vi "DIO card.vi"(8 "error in (no error)":errorcluster, 11 "Node Ptr":T4 format="%.0x") -> (0 "error out":errorcluster)   [LabVIEW 2014, in "SLSC configuration System Explorer.lvlib"]
uses:
  SLSC configuration System Explorer.lvlib
  <vilib>/NI Veristand/Custom Device API/Custom Device Item Ref.ctl
  Example/DIO Board/DIO Line Config.ctl
  Type Defs/Card Position.ctl
  Example/SPI Utility/Slot #.ctl
  Shared/Constants.vi
  <vilib>/NI Veristand/Custom Device API/Get Item Property (U16).vi
  <vilib>/NI Veristand/Custom Device API/Set Item Property (U16).vi
  <vilib>/NI Veristand/Custom Device API/Custom Device API.lvlib
  Shared/SLSC configuration Shared.lvlib
panel:
  in  "Card Position":T1 {"Slot #" max=16}
  in  "Logic Threshold (%) 3":u8 caption="Logic Threshold (%)"
  in  "DIO Line Config 3":T3=[FALSE, FALSE, FALSE, FALSE, FALSE, FALSE, FALSE, FALSE]
  in  "Header 5":cluster{"Section Name":string}={"Section Name"="Bank 3 Settings"}
  in  "Logic Threshold (%) 2":u8 caption="Logic Threshold (%)"
  in  "DIO Line Config 2":T3=[FALSE, FALSE, FALSE, FALSE, FALSE, FALSE, FALSE, FALSE]
  in  "Header 4":cluster{"Section Name":string}={"Section Name"="Bank 2 Settings"}
  in  "Header 3":cluster{"Section Name":string}={"Section Name"="Bank 1 Settings"}
  in  "Logic Threshold (%) 1":u8 caption="Logic Threshold (%)"
  in  "DIO Line Config 1":T3=[FALSE, FALSE, FALSE, FALSE, FALSE, FALSE, FALSE, FALSE]
  in  "Header 2":cluster{"Section Name":string}={"Section Name"="Bank 0 Settings"}
  in  "Logic Threshold (%) 0":u8 caption="Logic Threshold (%)"
  in  "DIO Line Config 0":T3=[FALSE, FALSE, FALSE, FALSE, FALSE, FALSE, FALSE, FALSE]
  in  "Header":cluster{"Section Name":string}={"Section Name"="DIO Card Settings"}
  in  "Description":string
  in  "Name":string
  # "Line 9"
  # "Line 10"
  # "Line 11"
  # "Line 12"
  # "Line 13"
  # "Line 14"
  # "Line 15"
  # "Line 16"
  # "Line 17"
  # "Line 18"
  # "Line 19"
  # "Line 20"
  # "Line 21"
  # "Line 22"
  # "Line 23"
  # "Line 24"
  # "Line 25"
  # "Line 26"
  # "Line 27"
  # "Line 28"
  # "Line 29"
  # "Line 30"
  # "Line 31"
  # "Line 32"
  # "Line 1"
  # "Line 2"
  # "Line 3"
  # "Line 4"
  # "Line 5"
  # "Line 6"
  # "Line 7"
  # "Line 8"
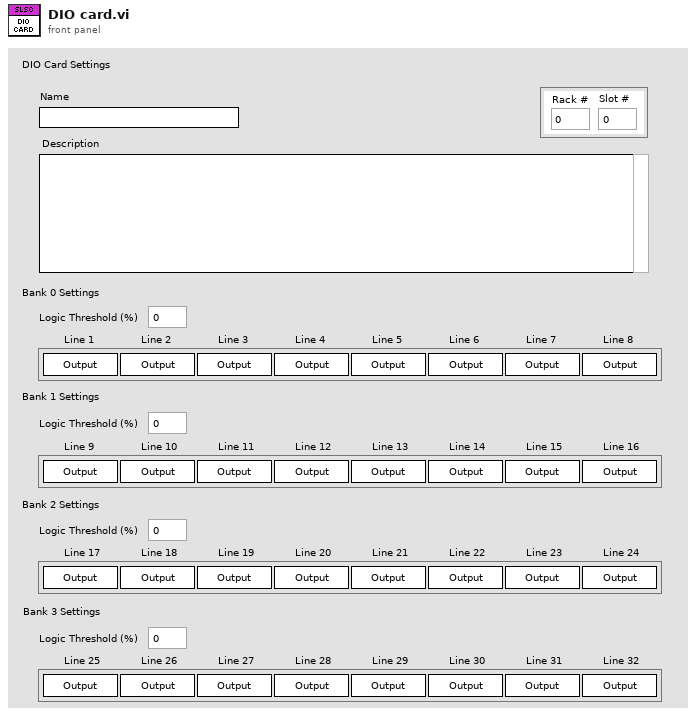
[diagram p1: front panel]
types:
  T1 = typedef "SLSC configuration Shared.lvlib/Card Position.ctl" = cluster{"Rack #":u8, "Slot #":T2}
  T2 = typedef "SLSC configuration Shared.lvlib/Slot #.ctl" = u8
  T3 = typedef "SLSC configuration Shared.lvlib/DIO Line Config.ctl" = bool[]
  T4 = typedef "Custom Device API.lvlib/Custom Device Item Ref.ctl" = u64
  T5 = typedef "Custom Device API.lvlib/Custom Device Commands.ctl" = enum16{"Default", "Item renamed", "Shutdown", "Dynamic button pressed"}
  T6 = typedef "Custom Device API.lvlib/Custom Device Item Info.ctl" = cluster{"Name":string, "Is Channel":bool, "GUID":string, "Is Waveform":bool}
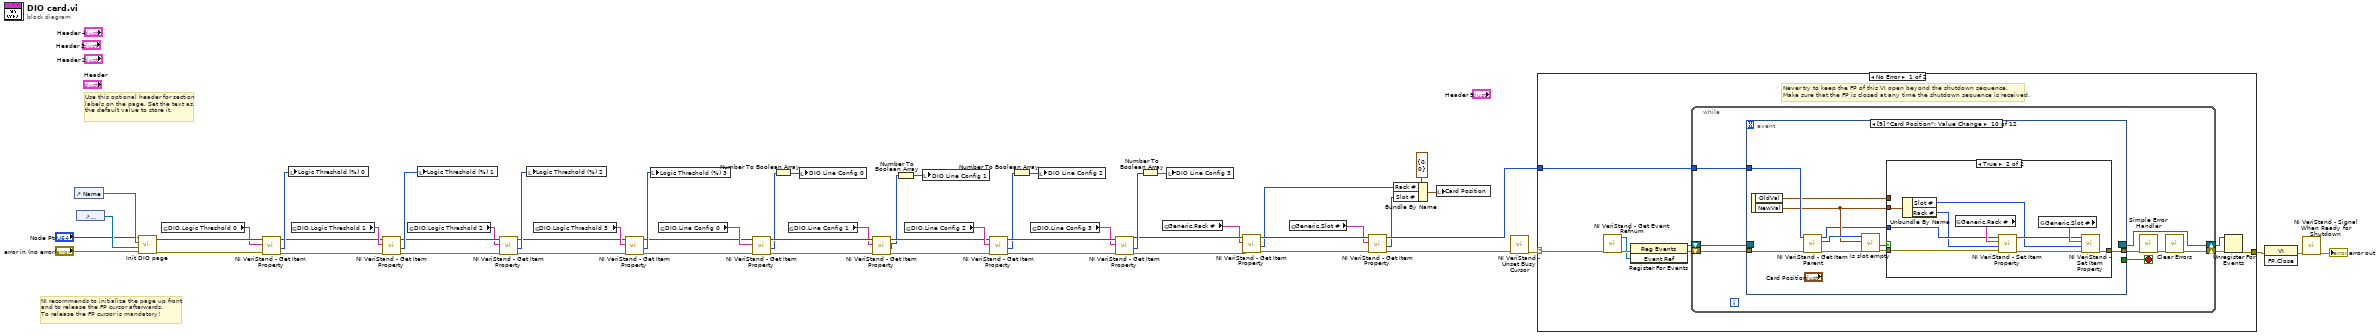
[diagram p0: block diagram]
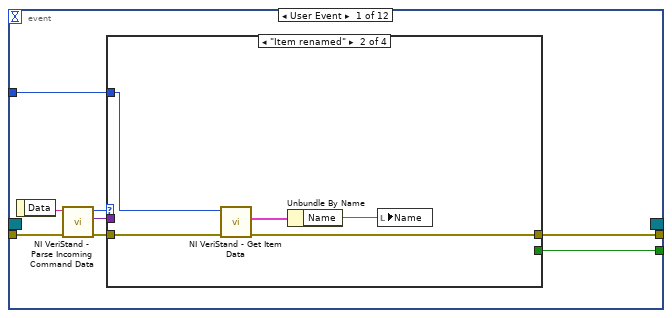
[diagram p2: hidden frame]
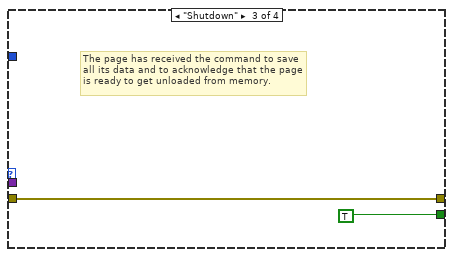
[diagram p4: hidden frame]
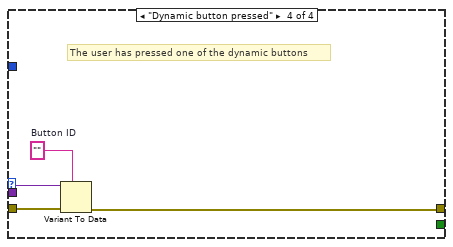
[diagram p5: hidden frame]
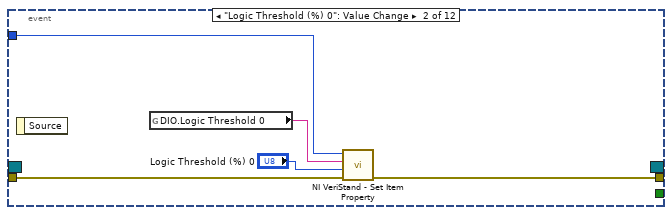
[diagram p6: hidden frame]
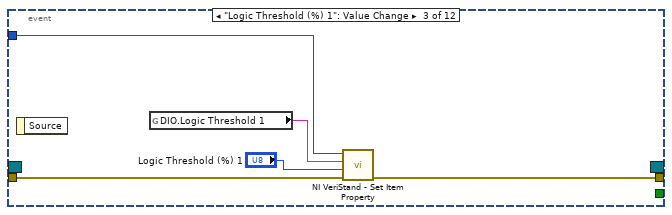
[diagram p7: hidden frame]
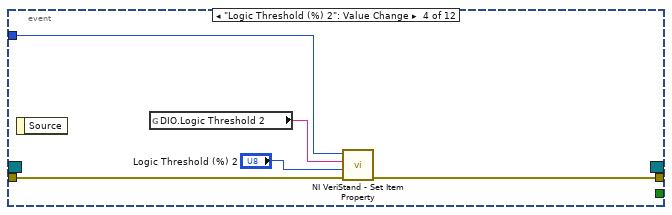
[diagram p8: hidden frame]
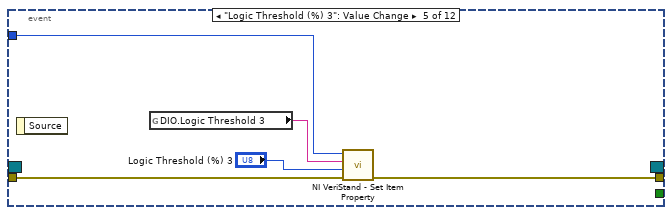
[diagram p9: hidden frame]
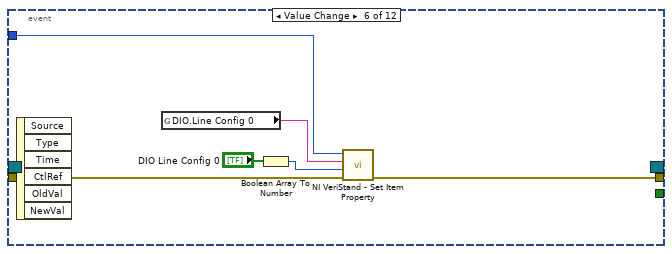
[diagram p10: hidden frame]
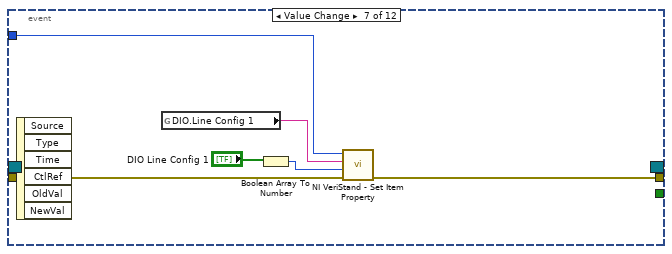
[diagram p11: hidden frame]
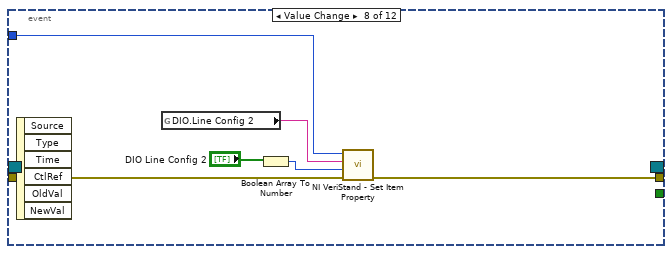
[diagram p12: hidden frame]
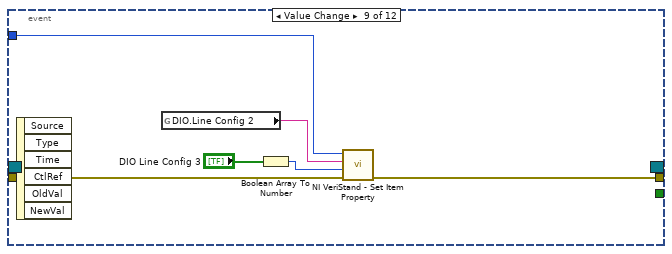
[diagram p13: hidden frame]
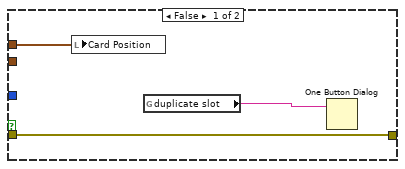
[diagram p14: hidden frame]
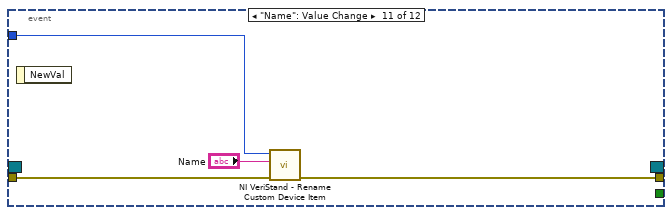
[diagram p15: hidden frame]
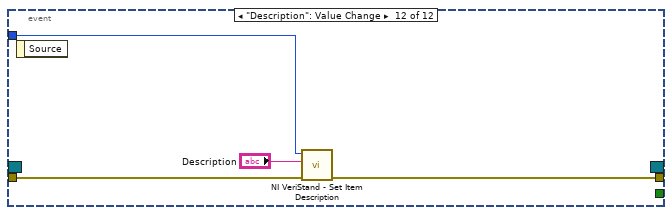
[diagram p16: hidden frame]
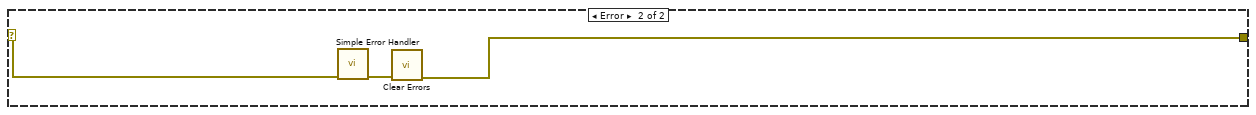
[diagram p17: hidden frame]
diagram:
  # "Use this optional header for section labels on the page. Set the text as the default value to store it."
  # "NI recommends to initialize the page up front\nand to release the FP cursor afterwards.\nTo release the FP cursor is mandatory!"
  n1 = control-ref of="Name"() -> (w52:refnum<vi>)
  n2 = control-ref of="Description"() -> (w51:refnum<vi>)
  n3 = call "Init DIO page.vi"("error in (no error)"="error in (no error)", "Description"=w51, "Name"=w52, "Node Ptr"="Node Ptr") -> ("error out"=w48:errorcluster, "Node Ptr out"=w47:T4)  [unwired: 6 in]
  n4 = global read "Constants.vi" "DIO.Logic Threshold 0"() -> (w45:string)
  n5 = call-poly <vilib>:"NI VeriStand - Get Item Property.vi"("error in (no error)"=w48, "Property Name"=w45, "Item Ref in"=w47) -> ("error out"=w42:errorcluster, "Value"=w46:u16, "Item Ref out"=w41:T4)  [unwired: 5 in, 1 out]
  n6 = local write "Logic Threshold (%) 0"(w46) -> ()
  n7 = global read "Constants.vi" "DIO.Logic Threshold 1"() -> (w44:string)
  n8 = call-poly <vilib>:"NI VeriStand - Get Item Property.vi"("error in (no error)"=w42, "Property Name"=w44, "Item Ref in"=w41) -> ("error out"=w39:errorcluster, "Value"=w43:u16, "Item Ref out"=w38:T4)  [unwired: 5 in, 1 out]
  n9 = global read "Constants.vi" "DIO.Logic Threshold 2"() -> (w37:string)
  n10 = local write "Logic Threshold (%) 1"(w43) -> ()
  n11 = call-poly <vilib>:"NI VeriStand - Get Item Property.vi"("error in (no error)"=w39, "Property Name"=w37, "Item Ref in"=w38) -> ("error out"=w34:errorcluster, "Value"=w40:u16, "Item Ref out"=w33:T4)  [unwired: 5 in, 1 out]
  n12 = local write "Logic Threshold (%) 2"(w40) -> ()
  n13 = global read "Constants.vi" "DIO.Logic Threshold 3"() -> (w36:string)
  n14 = call-poly <vilib>:"NI VeriStand - Get Item Property.vi"("error in (no error)"=w34, "Property Name"=w36, "Item Ref in"=w33) -> ("error out"=w21:errorcluster, "Value"=w35:u16, "Item Ref out"=w20:T4)  [unwired: 5 in, 1 out]
  n15 = local write "Logic Threshold (%) 3"(w35) -> ()
  n16 = global read "Constants.vi" "DIO.Line Config 0"() -> (w23:string)
  n17 = call-poly <vilib>:"NI VeriStand - Get Item Property.vi"("error in (no error)"=w21, "Property Name"=w23, "Item Ref in"=w20) -> ("error out"=w25:errorcluster, "Value"=w22:u16, "Item Ref out"=w26:T4)  [unwired: 5 in, 1 out]
  n18 = Number To Boolean Array(number=w22) -> (Boolean array=w19:bool[])
  n19 = global read "Constants.vi" "DIO.Line Config 1"() -> (w24:string)
  n20 = local write "DIO Line Config 0"(w19) -> ()
  n21 = call-poly <vilib>:"NI VeriStand - Get Item Property.vi"("error in (no error)"=w25, "Property Name"=w24, "Item Ref in"=w26) -> ("error out"=w27:errorcluster, "Value"=w17:u16, "Item Ref out"=w28:T4)  [unwired: 5 in, 1 out]
  n22 = Number To Boolean Array(number=w17) -> (Boolean array=w18:bool[])
  n23 = global read "Constants.vi" "DIO.Line Config 2"() -> (w29:string)
  n24 = local write "DIO Line Config 1"(w18) -> ()
  n25 = call-poly <vilib>:"NI VeriStand - Get Item Property.vi"("error in (no error)"=w27, "Property Name"=w29, "Item Ref in"=w28) -> ("error out"=w31:errorcluster, "Value"=w15:u16, "Item Ref out"=w32:T4)  [unwired: 5 in, 1 out]
  n26 = Number To Boolean Array(number=w15) -> (Boolean array=w16:bool[])
  n27 = global read "Constants.vi" "DIO.Line Config 3"() -> (w30:string)
  n28 = local write "DIO Line Config 2"(w16) -> ()
  n29 = call-poly <vilib>:"NI VeriStand - Get Item Property.vi"("error in (no error)"=w31, "Property Name"=w30, "Item Ref in"=w32) -> ("error out"=w9:errorcluster, "Value"=w13:u16, "Item Ref out"=w8:T4)  [unwired: 5 in, 1 out]
  n30 = Number To Boolean Array(number=w13) -> (Boolean array=w14:bool[])
  n31 = global read "Constants.vi" "Generic.Rack #"() -> (w7:string)
  n32 = local write "DIO Line Config 3"(w14) -> ()
  n33 = call-poly <vilib>:"NI VeriStand - Get Item Property.vi"("error in (no error)"=w9, "Property Name"=w7, "Item Ref in"=w8) -> ("error out"=w11:errorcluster, "Value"=w3:u16, "Item Ref out"=w12:T4)  [unwired: 5 in, 1 out]
  n34 = global read "Constants.vi" "Generic.Slot #"() -> (w10:string)
  n35 = call-poly <vilib>:"NI VeriStand - Get Item Property.vi"("error in (no error)"=w11, "Property Name"=w10, "Item Ref in"=w12) -> ("error out"=w6:errorcluster, "Value"=w2:u16, "Item Ref out"=w5:T4)  [unwired: 5 in, 1 out]
  n36 = Bundle By Name(cluster=T1 {"Rack #"=0, "Slot #"=0} ("Card Position"), "Rack #"=w3, "Slot #"=w2) -> (w1:T1)
  n37 = local write "Card Position"(w1) -> ()
  n38 = call <vilib>:"NI VeriStand - Unset Busy Cursor.vi"("error in (no error)"=w6) -> ("error out"=w53:errorcluster)  [unwired: 10 out]
  n39 = case shown="No Error" w53 {
    selector: w53 -> [w58 w171]
    tunnel: [w62 w169] -> w56
    tunnel: w5 -> [w57 _]
    frame No Error {
      # "Never try to keep the FP of this VI open beyond the shutdown sequence.\nMake sure that the FP is closed at any time the shutdown sequence is received."
      n40 = call <vilib>:"NI VeriStand - Get Event Refnum.vi"("error in (no error)"=w58) -> ("error out"=w65:errorcluster, "Event Ref"=w61:refnum<user-event>)  [unwired: 9 out]
      n41 = register-events(error in=w65, w61) -> (reference out=w59:refnum<event-registration>, error out=w60:errorcluster)  [unwired: 1 in]
      n42 = while {
        shift-right: [w67] -> w63
        shift-left: w60 -> [w72]
        shift-right: [w73] -> w64
        shift-left: w59 -> [w71]
        tunnel: w57 -> [w66]
        stop <- w70 stop-if-true
        n43 = event shown="[9] \"Card Position\": Value Change" {
          selector: w71 -> [_ _ _ _ _ _ _ _ _ _ _ _]
          dyn-events: [_ _ _ _ _ _ _ _ _ _ _ _] -> w73
          timeout: _ -> [_ _ _ _ _ _ _ _ _ _ _ _]
          tunnel: w72 -> [w81 w98 w103 w108 w113 w119 w125 w131 w137 w146 w164 w168]
          tunnel: [w77 _ _ _ _ _ _ _ _ _ _ _] -> w70
          tunnel: [w76 w97 w102 w107 w112 w118 w124 w130 w136 w147 w163 w167] -> w69
          tunnel: w66 -> [w74 w94 w99 w104 w109 w114 w120 w126 w132 w145 w161 w165]
          event User Event {
            n44 = event-data() -> ("Data"=w80:string)  [unwired: 1 out]
            n45 = call <vilib>:"NI VeriStand - Parse Incoming Command Data.vi"("error in (no error)"=w81, "Incoming data"=w80) -> ("error out"=w79:errorcluster, "Outgoing data"=w75:variant, "Action"=w78:T5)  [unwired: 7 out]
            n46 = case shown="\"Item renamed\"" w78 {
              tunnel: w79 -> [w82 w87 w88 w93]
              tunnel: [_ _ TRUE _] -> w77
              tunnel: [w82 w85 w88 w90] -> w76
              tunnel: w75 -> [_ _ _ w92]
              tunnel: w74 -> [_ w83 _ _]
              frame "Default", Default {
              }
              frame "Item renamed" {
                n47 = call <vilib>:"NI VeriStand - Get Item Data.vi"("error in (no error)"=w87, "Item Ref in"=w83) -> ("error out"=w85:errorcluster, "Item Info"=w86:T6)  [unwired: 8 out]
                n48 = Unbundle By Name(w86) -> ("Name"=w84:string)
                n49 = local write "Name"(w84) -> ()
              }
              frame "Shutdown" {
                # "The page has received the command to save all its data and to acknowledge that the page is ready to get unloaded from memory."
              }
              frame "Dynamic button pressed" {
                w91 = ""  # Button ID
                # "The user has pressed one of the dynamic buttons"
                n50 = Variant To Data(error in=w93, type=w91, Variant=w92) -> (error out=w90:errorcluster)  [unwired: 1 out]
              }
            }
          }
          event "Logic Threshold (%) 0": Value Change {
            n51 = event-data() -> ()  [unwired: 2 out]
            n52 = global read "Constants.vi" "DIO.Logic Threshold 0"() -> (w95:string)
            n53 = call-poly <vilib>:"NI VeriStand - Set Item Property.vi"("error in (no error)"=w98, "Value"="Logic Threshold (%) 0", "Property Name"=w95, "Item Ref in"=w94) -> ("error out"=w97:errorcluster)  [unwired: 5 in, 2 out]
          }
          event "Logic Threshold (%) 1": Value Change {
            n54 = event-data() -> ()  [unwired: 2 out]
            n55 = global read "Constants.vi" "DIO.Logic Threshold 1"() -> (w101:string)
            n56 = call-poly <vilib>:"NI VeriStand - Set Item Property.vi"("error in (no error)"=w103, "Value"="Logic Threshold (%) 1", "Property Name"=w101, "Item Ref in"=w99) -> ("error out"=w102:errorcluster)  [unwired: 5 in, 2 out]
          }
          event "Logic Threshold (%) 2": Value Change {
            n57 = event-data() -> ()  [unwired: 2 out]
            n58 = global read "Constants.vi" "DIO.Logic Threshold 2"() -> (w106:string)
            n59 = call-poly <vilib>:"NI VeriStand - Set Item Property.vi"("error in (no error)"=w108, "Value"="Logic Threshold (%) 2", "Property Name"=w106, "Item Ref in"=w104) -> ("error out"=w107:errorcluster)  [unwired: 5 in, 2 out]
          }
          event "Logic Threshold (%) 3": Value Change {
            n60 = event-data() -> ()  [unwired: 2 out]
            n61 = global read "Constants.vi" "DIO.Logic Threshold 3"() -> (w111:string)
            n62 = call-poly <vilib>:"NI VeriStand - Set Item Property.vi"("error in (no error)"=w113, "Value"="Logic Threshold (%) 3", "Property Name"=w111, "Item Ref in"=w109) -> ("error out"=w112:errorcluster)  [unwired: 5 in, 2 out]
          }
          event Value Change {
            n63 = event-data() -> ()  [unwired: 7 out]
            n64 = global read "Constants.vi" "DIO.Line Config 0"() -> (w117:string)
            n65 = Boolean Array To Number(Boolean array="DIO Line Config 0") -> (number=w115:u8)
            n66 = call-poly <vilib>:"NI VeriStand - Set Item Property.vi"("error in (no error)"=w119, "Value"=w115, "Property Name"=w117, "Item Ref in"=w114) -> ("error out"=w118:errorcluster)  [unwired: 5 in, 2 out]
          }
          event Value Change {
            n67 = event-data() -> ()  [unwired: 7 out]
            n68 = global read "Constants.vi" "DIO.Line Config 1"() -> (w123:string)
            n69 = Boolean Array To Number(Boolean array="DIO Line Config 1") -> (number=w122:u8)
            n70 = call-poly <vilib>:"NI VeriStand - Set Item Property.vi"("error in (no error)"=w125, "Value"=w122, "Property Name"=w123, "Item Ref in"=w120) -> ("error out"=w124:errorcluster)  [unwired: 5 in, 2 out]
          }
          event Value Change {
            n71 = event-data() -> ()  [unwired: 7 out]
            n72 = global read "Constants.vi" "DIO.Line Config 2"() -> (w129:string)
            n73 = Boolean Array To Number(Boolean array="DIO Line Config 2") -> (number=w128:u8)
            n74 = call-poly <vilib>:"NI VeriStand - Set Item Property.vi"("error in (no error)"=w131, "Value"=w128, "Property Name"=w129, "Item Ref in"=w126) -> ("error out"=w130:errorcluster)  [unwired: 5 in, 2 out]
          }
          event Value Change {
            n75 = event-data() -> ()  [unwired: 7 out]
            n76 = global read "Constants.vi" "DIO.Line Config 2"() -> (w135:string)
            n77 = Boolean Array To Number(Boolean array="DIO Line Config 3") -> (number=w134:u8)
            n78 = call-poly <vilib>:"NI VeriStand - Set Item Property.vi"("error in (no error)"=w137, "Value"=w134, "Property Name"=w135, "Item Ref in"=w132) -> ("error out"=w136:errorcluster)  [unwired: 5 in, 2 out]
          }
          event Value Change {
            n79 = event-data() -> ("OldVal"=w138:T1, "NewVal"=w140:T1)  [unwired: 1 out]
            n80 = call <vilib>:"NI VeriStand - Get Item Parent.vi"("error in (no error)"=w146, "Item Ref in"=w145) -> ("error out"=w144:errorcluster, "Parent Ref"=w143:T4, "Item Ref out"=w139:T4)  [unwired: 6 in, 1 out]
            n81 = call "Is slot empty.vi"("error in (no error)"=w144, "Card Position"=w140, "Devcie Ref in"=w143) -> ("error out"=w141:errorcluster, "Empty?"=w142:bool)  [unwired: 6 in, 1 out]
            n82 = case shown="True" w142 {
              tunnel: [w150 w154] -> w147
              tunnel: w141 -> [w150 w159]
              tunnel: w140 -> [_ w157]
              tunnel: w139 -> [_ w158]
              tunnel: w138 -> [w148 _]
              frame False {
                n83 = local write "Card Position"(w148) -> ()
                n84 = global read "Constants.vi" "duplicate slot"() -> (w149:string)
                n85 = One Button Dialog(message=w149) -> ()  [unwired: 1 in, 1 out]
              }
              frame True {
                n86 = Unbundle By Name(w157) -> ("Slot #"=w151:T2, "Rack #"=w152:u8)
                n87 = global read "Constants.vi" "Generic.Rack #"() -> (w160:string)
                n88 = call-poly <vilib>:"NI VeriStand - Set Item Property.vi"("error in (no error)"=w159, "Value"=w152, "Property Name"=w160, "Item Ref in"=w158) -> ("error out"=w155:errorcluster, "Item Ref out"=w153:T4)  [unwired: 5 in, 1 out]
                n89 = global read "Constants.vi" "Generic.Slot #"() -> (w156:string)
                n90 = call-poly <vilib>:"NI VeriStand - Set Item Property.vi"("error in (no error)"=w155, "Value"=w151, "Property Name"=w156, "Item Ref in"=w153) -> ("error out"=w154:errorcluster)  [unwired: 5 in, 2 out]
              }
            }
          }
          event "Name": Value Change {
            n91 = event-data() -> ()  [unwired: 2 out]
            n92 = call <vilib>:"NI VeriStand - Rename Custom Device Item.vi"("error in (no error)"=w164, "New Name"="Name", "Item Ref in"=w161) -> ("error out"=w163:errorcluster)  [unwired: 1 in, 7 out]
          }
          event "Description": Value Change {
            n93 = event-data() -> ()  [unwired: 2 out]
            n94 = call <vilib>:"NI VeriStand - Set Item Description.vi"("error in (no error)"=w168, "Description"="Description", "Item Ref in"=w165) -> ("error out"=w167:errorcluster)  [unwired: 8 out]
          }
        }
        n95 = call <vilib>:"Simple Error Handler.vi"("error in (no error)"=w69) -> ("error out"=w68:errorcluster)  [unwired: 1 in, 7 out]
        n96 = call <vilib>:"Clear Errors.vi"("error in (no error)"=w68) -> ("error out"=w67:errorcluster)  [unwired: 1 in, 5 out]
      }
      n97 = Unregister For Events(event registration refnum=w64, error in=w63) -> (error out=w62:errorcluster)
    }
    frame Error {
      n98 = call <vilib>:"Simple Error Handler.vi"("error in (no error)"=w171) -> ("error out"=w170:errorcluster)  [unwired: 1 in, 7 out]
      n99 = call <vilib>:"Clear Errors.vi"("error in (no error)"=w170) -> ("error out"=w169:errorcluster)  [unwired: 1 in, 5 out]
    }
  }
  n100 = invoke class="VI" method="FP.Close"(error in=w56) -> (error out=w55:errorcluster)  [unwired: 2 in, 2 out]
  n101 = call <vilib>:"NI VeriStand - Signal When Ready for Shutdown.vi"("error in (no error)"=w55) -> ("error out"=→"error out":errorcluster)  [unwired: 10 out]
